vi "get_update_owner_command.vi"(8 "error in (no error)":errorcluster, 11 "GenericImageProcessor.lvclass in":refnum<class "GenericImageProcessor.lvclass">) -> (0 "error out":errorcluster, 2 "update-owner command":refnum<class "GenericImageProcessorChangedCommand.lvclass">, 3 "GenericImageProcessor.lvclass out":refnum<class "GenericImageProcessor.lvclass">)   [LabVIEW 2010, in "GenericImageProcessor.lvclass"]
uses:
  GenericImageProcessor.lvclass
  Command/GenericImageProcessorChangedCommand/GenericImageProcessorChangedCommand/GenericImageProcessorChangedCommand.lvclass
  GenericImageProcessor.lvclass/GenericImageProcessor.ctl
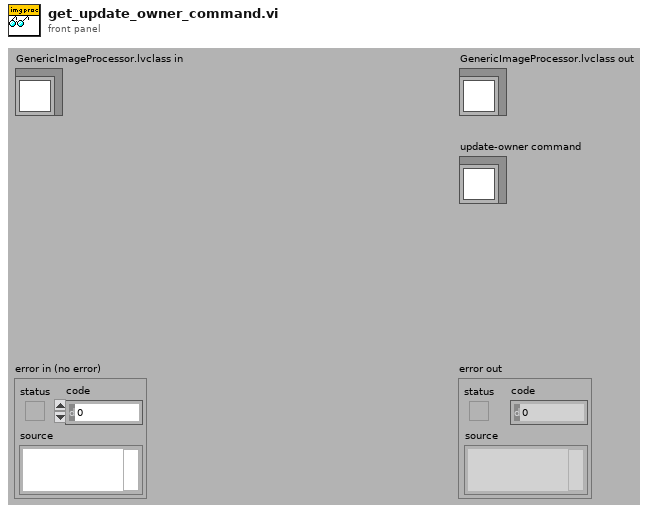
[diagram p1: front panel]
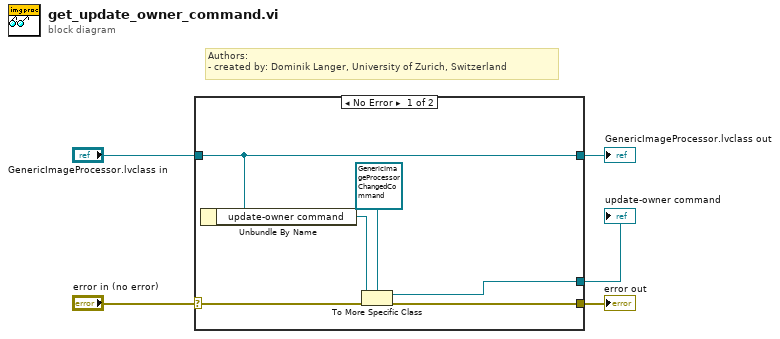
[diagram p0: block diagram]
diagram:
  # "Authors: \n- created by: Dominik Langer, University of Zurich, Switzerland"
  n1 = case shown="No Error" "error in (no error)" {
    selector: "error in (no error)" -> [w8 w12]
    tunnel: [w6 w12] -> w4
    tunnel: [w11 w13] -> w2
    tunnel: "GenericImageProcessor.lvclass in" -> [w11 w13]
    tunnel: [w7 _] -> w1
    frame No Error {
      n2 = Unbundle By Name(w11) -> ("update-owner command"=w10:refnum<class "GenericCommand.lvclass">)
      n3 = To More Specific Class(target class=refnum<class "GenericImageProcessorChangedCommand.lvclass"> refnum ("GenericImageProcessorChangedCommand.lvclass"), reference=w10, error in=w8) -> (specific class reference=w7:refnum<class "GenericImageProcessorChangedCommand.lvclass">, error out=w6:errorcluster)
    }
    frame Error {
    }
  }
  "error out" <- w4
  "GenericImageProcessor.lvclass out" <- w2
  "update-owner command" <- w1
